vi "P2P_vst_ini.vi"(8 "error in (no error)":errorcluster, 11 "secnario config":T1={"devicess 2"=["IF_transiver_1", "IF_transiver_2"], "file paths"=[path "C:/Users/PXIe8108_Demo/Documents/CHAIM DATA/chaim/5785_sync_for_elbit/data/pdw_test_file.tdms", path "C:/Users/PXIe8108_Demo/Documents/CHAIM DATA/chaim/5785_sync_for_elbit/data/pdw_test_file.tdms", path "C:/Users/PXIe8108_Demo/Documents/CHAIM DATA/chaim/5785_sync_for_elbit/data/pdw_test_file.tdms", path "C:/Users/PXIe8108_Demo/Documents/CHAIM DATA/chaim/5785_sync_for_elbit/data/pdw_test_file.tdms"], "buffer size"=524288, "Fs  FPGA"=200000000.0, "SPC"=16.0, "center frequency (Hz) "=1000000000.0, "t clock ref"=[], "fpga rfe"=[], "tdms refs"=[], "niUsrpRio Session (out)"={"FPGA Interface"=refnum, "RIO Interface Number"=0, "Data Clock Rate"=0, "FPGA Data Clock Rate"=0, "Global Settings Register Bus"=refnum, "Radio 0 Settings Register Bus"=refnum, "Radio 1 Settings Register Bus"=refnum, "Radio Settings Bus Semaphore"=refnum, "DB Queues"=[], "Characterization Data Valid?"=FALSE, "EEPROM Header"={"Checksum"=0, "Product Code"=0, "Hardware Current Version"=0, "Hardware Oldest Compatible Version"=0, "EEPROM Map Current Version"=0, "EEPROM Map Oldest Compatible Version"=0, "User Password"="", "Pointer to Factory Header"=0, "Pointer to User Header"=0, "Recommended Interval"=0, "Number of Reserved Bytes"=9, "Number of Daughterboards"=0, "Daughterboard IDs"=[], "Daughterboard Serial Numbers"=[]}, "Device Data Header"={"Checksum"=0, "Number of Channels"=0, "Number of Gain Settings"=[], "Pointer to Characterization Data"=[], "Number of Reserved Bytes"=27, "Number of Frequencies"=[]}, "EEPROM Characterization Header"={"Checksum"=0, "Date"=timestamp(0 s since 1904-01-01), "Temperature"=0.0, "Misc. Info"="", "Pointer to Device Data Header"=0, "Number of Reserved Bytes"=28}, "Characterization Data"=[], "FPGA Current Version"=0, "FPGA Oldest Compatible Version"=0, "Fixed Logic Current Version"=0, "Fixed Logic Oldest Compatible Version"=0, "FPGA Radio Settings Bus Current Version"=0, "FPGA Radio Settings Bus Oldest Compatible Version"=0, "FPGA Board Config Current Version"=0, "FPGA Board Config Oldest Compatible Version"=0, "Daughterboard Clock Rate"=0, "daughterboard configuration session handles"=[]}, "RF gain "=10, "mode"=0, "vst_device"=[]} {"mode" scale=0.0..2.0; "RF gain" min=0 max=31 step=1; "niUsrpRio Session (out)"."Daughterboard Clock Rate" format="%#.3pHz"; "niUsrpRio Session (out)"."FPGA Data Clock Rate" format="%#.3pHz"; "niUsrpRio Session (out)"."Data Clock Rate" format="%#.3pHz"; "niUsrpRio Session (out)"."Characterization Data"."Frequencies [Hz]" format="%#_6p"; "niUsrpRio Session (out)"."EEPROM Characterization Header"."Pointer to Device Data Header" format="%x"; "niUsrpRio Session (out)"."EEPROM Characterization Header"."Checksum" format="%x"; "niUsrpRio Session (out)"."Device Data Header"."Pointer to Characterization Data" format="%x"; "niUsrpRio Session (out)"."Device Data Header"."Checksum" format="%x"; "niUsrpRio Session (out)"."EEPROM Header"."Pointer to User Header" format="%x"; "niUsrpRio Session (out)"."EEPROM Header"."Pointer to Factory Header" format="%x"; "niUsrpRio Session (out)"."EEPROM Header"."Product Code" format="%x"; "niUsrpRio Session (out)"."EEPROM Header"."Checksum" format="%x"; "center frequency (Hz)" format="%#.8p"; "buffer size" step=512}) -> (0 "error out":errorcluster, 3 "secnario config":T1={"devicess 2"=["IF_transiver_1", "IF_transiver_2"], "file paths"=[path "C:/Users/PXIe8108_Demo/Documents/CHAIM DATA/chaim/5785_sync_for_elbit/data/pdw_test_file.tdms", path "C:/Users/PXIe8108_Demo/Documents/CHAIM DATA/chaim/5785_sync_for_elbit/data/pdw_test_file.tdms", path "C:/Users/PXIe8108_Demo/Documents/CHAIM DATA/chaim/5785_sync_for_elbit/data/pdw_test_file.tdms", path "C:/Users/PXIe8108_Demo/Documents/CHAIM DATA/chaim/5785_sync_for_elbit/data/pdw_test_file.tdms"], "buffer size"=524288, "Fs  FPGA"=200000000.0, "SPC"=16.0, "center frequency (Hz) "=1000000000.0, "t clock ref"=[], "fpga rfe"=[], "tdms refs"=[], "niUsrpRio Session (out)"={"FPGA Interface"=refnum, "RIO Interface Number"=0, "Data Clock Rate"=0, "FPGA Data Clock Rate"=0, "Global Settings Register Bus"=refnum, "Radio 0 Settings Register Bus"=refnum, "Radio 1 Settings Register Bus"=refnum, "Radio Settings Bus Semaphore"=refnum, "DB Queues"=[], "Characterization Data Valid?"=FALSE, "EEPROM Header"={"Checksum"=0, "Product Code"=0, "Hardware Current Version"=0, "Hardware Oldest Compatible Version"=0, "EEPROM Map Current Version"=0, "EEPROM Map Oldest Compatible Version"=0, "User Password"="", "Pointer to Factory Header"=0, "Pointer to User Header"=0, "Recommended Interval"=0, "Number of Reserved Bytes"=9, "Number of Daughterboards"=0, "Daughterboard IDs"=[], "Daughterboard Serial Numbers"=[]}, "Device Data Header"={"Checksum"=0, "Number of Channels"=0, "Number of Gain Settings"=[], "Pointer to Characterization Data"=[], "Number of Reserved Bytes"=27, "Number of Frequencies"=[]}, "EEPROM Characterization Header"={"Checksum"=0, "Date"=timestamp(0 s since 1904-01-01), "Temperature"=0.0, "Misc. Info"="", "Pointer to Device Data Header"=0, "Number of Reserved Bytes"=28}, "Characterization Data"=[], "FPGA Current Version"=0, "FPGA Oldest Compatible Version"=0, "Fixed Logic Current Version"=0, "Fixed Logic Oldest Compatible Version"=0, "FPGA Radio Settings Bus Current Version"=0, "FPGA Radio Settings Bus Oldest Compatible Version"=0, "FPGA Board Config Current Version"=0, "FPGA Board Config Oldest Compatible Version"=0, "Daughterboard Clock Rate"=0, "daughterboard configuration session handles"=[]}, "RF gain "=10, "mode"=0, "vst_device"=[]} {"mode" scale=0.0..2.0; "RF gain" min=0 max=31 step=1; "niUsrpRio Session (out)"."Daughterboard Clock Rate" format="%#.3pHz"; "niUsrpRio Session (out)"."FPGA Data Clock Rate" format="%#.3pHz"; "niUsrpRio Session (out)"."Data Clock Rate" format="%#.3pHz"; "niUsrpRio Session (out)"."Characterization Data"."Frequencies [Hz]" format="%#_6p"; "niUsrpRio Session (out)"."EEPROM Characterization Header"."Pointer to Device Data Header" format="%x"; "niUsrpRio Session (out)"."EEPROM Characterization Header"."Checksum" format="%x"; "niUsrpRio Session (out)"."Device Data Header"."Pointer to Characterization Data" format="%x"; "niUsrpRio Session (out)"."Device Data Header"."Checksum" format="%x"; "niUsrpRio Session (out)"."EEPROM Header"."Pointer to User Header" format="%x"; "niUsrpRio Session (out)"."EEPROM Header"."Pointer to Factory Header" format="%x"; "niUsrpRio Session (out)"."EEPROM Header"."Product Code" format="%x"; "niUsrpRio Session (out)"."EEPROM Header"."Checksum" format="%x"; "center frequency (Hz)" format="%#.8p"; "buffer size" step=512})   [LabVIEW 2021]
uses:
  <vilib>/rvi/interface/nirviMethod/nirviMethod.xnode
  <vilib>/rvi/errors/niLvFpgaMergeErrorWithErrorCode.vi
  <vilib>/rvi/interface/nirviReadWriteControl/nirviReadWriteControl.xnode
  <vilib>/rvi/interface/nirviOpenFPGA/nirviOpenFPGA.xnode
  <instrlib>/niRFSG/niRFSG.llb/niRFSG Ref Clock Sources.ctl
  <instrlib>/niRFSG/niRFSG.llb/niRFSG Configure Start Trigger P2P Endpoint Fullness.vi
  <vilib>/FPGAPlugInAG/Dynamic/niLvFpga_StopFifo_Dynamic.vi
  <vilib>/FPGAPlugInAG/Dynamic/niLvFpga_ConfigureFifo_Dynamic.vi
  NiFpgaLv.dll
  <vilib>/Utility/error.llb/Error Cluster From Error Code.vi
  <vilib>/rvi/interface/Simulation/niFpgaSimulationCallBeginRW.vi
  <vilib>/rvi/errors/niLvFpgaAdjustHostInterfaceError.vi
  Users/PXIe8108_Demo/Documents/CHAIM DATA/chaim/5785_sync_for_elbit/tx_pulse/EMEA_ADG_EW_secnario_TX_PDW_to_pulses/FPGA Bitfiles/P2P_Pulse.lvbitx
  Users/PXIe8108_Demo/Documents/CHAIM DATA/chaim/5785_sync_for_elbit/tx_pulse/EMEA_ADG_EW_secnario_TX_PDW_to_pulses/fpga/5785_p2p_IQ_gen.vi
  <vilib>/FPGAPlugInAG/PXIe-5785 (KU060)/niLvFpga_Open_PXIe-5785 (KU060).vi
  <vilib>/rvi/interface/common/dynamic/niFpgaDynamicAddResources.vi
  <vilib>/userDefined/High Color/nirio_resource_hc.ctl
  secnario config.ctl
  Program Files/National Instruments/LabVIEW 2022/instr.lib/_niInstr/Register Bus/v0/Host/Private/Session Data.ctl
  Program Files/National Instruments/LabVIEW 2022/instr.lib/_niInstr/Register Bus/v0/Host/niInstr Register Bus v0 Host.lvlib
  Program Files/National Instruments/LabVIEW 2022/instr.lib/_niInstr/Register Bus/v0/Host/Public/Register Bus Session.ctl
  Program Files/National Instruments/LabVIEW 2022/instr.lib/niUsrpRio/Config/v1/Host/Public/EEPROM Header.ctl
  Program Files/National Instruments/LabVIEW 2022/instr.lib/niUsrpRio/Config/v1/Host/niUsrpRio Config v1 Host.lvlib
  Program Files/National Instruments/LabVIEW 2022/instr.lib/niUsrpRio/Config/v1/Host/Public/EEPROM Device Data Header.ctl
  Program Files/National Instruments/LabVIEW 2022/instr.lib/niUsrpRio/Config/v1/Host/Public/EEPROM Characterization Header.ctl
  Program Files/National Instruments/LabVIEW 2022/instr.lib/niUsrpRio/Config/v1/Host/Public/IQ Imbalance.ctl
  Program Files/National Instruments/LabVIEW 2022/instr.lib/niUsrpRio/Config/v1/Host/Public/Characterization Data.ctl
  Program Files/National Instruments/LabVIEW 2022/instr.lib/niUsrpRio/Config/v1/Host/Private/Antenna Configuration.ctl
  Program Files/National Instruments/LabVIEW 2022/instr.lib/niUsrpRio/Config/v1/Host/Private/ATR state data.ctl
  Program Files/National Instruments/LabVIEW 2022/instr.lib/niUsrpRio/Config/v1/Host/Private/CPLD Power Mode.ctl
  Program Files/National Instruments/LabVIEW 2022/instr.lib/niUsrpRio/Config/v1/Host/Private/Daughterboard Data.ctl
  Program Files/National Instruments/LabVIEW 2022/instr.lib/niUsrpRio/Config/v1/Host/Private/DB Queue Reference.ctl
  Program Files/National Instruments/LabVIEW 2022/instr.lib/niUsrpRio/Config/v1/Host/Public/niUsrpRio Session.ctl
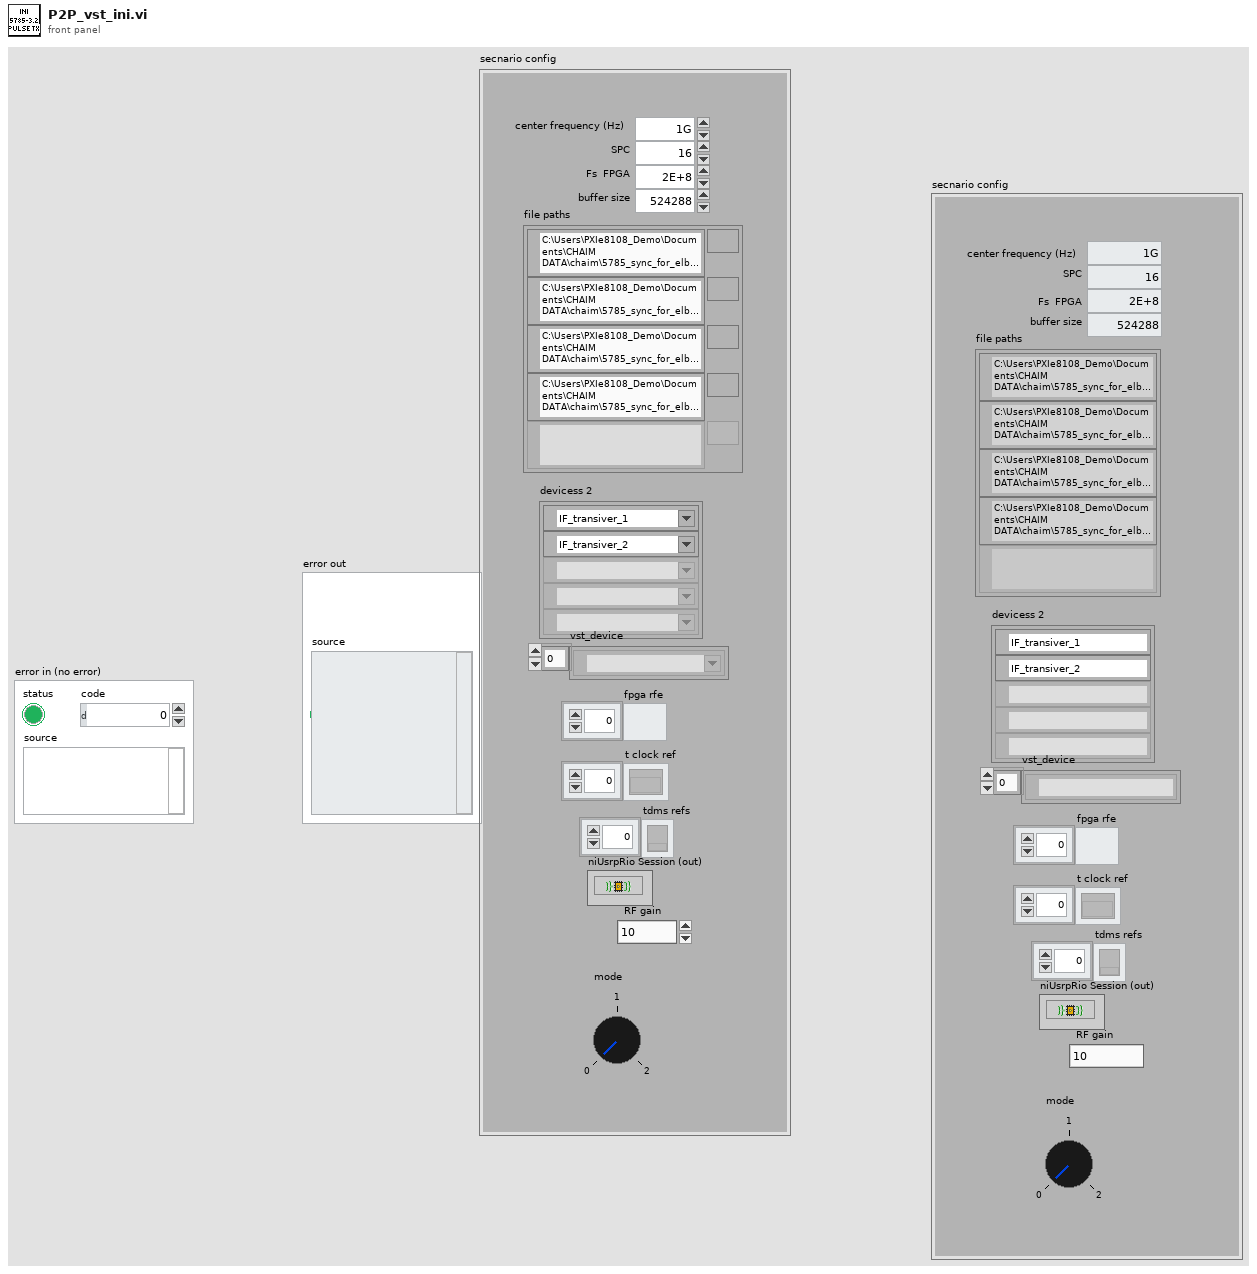
[diagram p1: front panel]
types:
  T1 = typedef "secnario config.ctl" = cluster{"devicess 2":T2[], "file paths":path[], "buffer size":u32, "Fs  FPGA":dbl, "SPC":dbl, "center frequency (Hz) ":dbl, "t clock ref":refnum<k20>[], "fpga rfe":refnum<k20>[], "tdms refs":refnum<k34>[], "niUsrpRio Session (out)":T3, "RF gain ":i32, "mode":u8, "vst_device":refnum<k15>[]}
  T2 = typedef "nirio_resource_hc.ctl" = tag
  T3 = typedef "niUsrpRio Config v1 Host.lvlib/niUsrpRio Session.ctl" = cluster{"FPGA Interface":refnum<k20>, "RIO Interface Number":u32, "Data Clock Rate":u32, "FPGA Data Clock Rate":u32, "Global Settings Register Bus":T4, "Radio 0 Settings Register Bus":T4, "Radio 1 Settings Register Bus":T4, "Radio Settings Bus Semaphore":T5, "DB Queues":T6[], "Characterization Data Valid?":bool, "EEPROM Header":T7, "Device Data Header":T8, "EEPROM Characterization Header":T9, "Characterization Data":T10[], "FPGA Current Version":u32, "FPGA Oldest Compatible Version":u32, "Fixed Logic Current Version":u32, "Fixed Logic Oldest Compatible Version":u32, "FPGA Radio Settings Bus Current Version":u32, "FPGA Radio Settings Bus Oldest Compatible Version":u32, "FPGA Board Config Current Version":u32, "FPGA Board Config Oldest Compatible Version":u32, "Daughterboard Clock Rate":u32, "daughterboard configuration session handles":u64[]}
  T4 = typedef "niInstr Register Bus v0 Host.lvlib/Register Bus Session.ctl" = refnum<queue>
  T5 = typedef "Semaphore RefNum" = refnum<k1>
  T6 = typedef "niUsrpRio Config v1 Host.lvlib/DB Queue Reference.ctl" = refnum<queue>
  T7 = typedef "niUsrpRio Config v1 Host.lvlib/EEPROM Header.ctl" = cluster{"Checksum":u32, "Product Code":u16, "Hardware Current Version":u16, "Hardware Oldest Compatible Version":u16, "EEPROM Map Current Version":u16, "EEPROM Map Oldest Compatible Version":u16, "User Password":string, "Pointer to Factory Header":u32, "Pointer to User Header":u32, "Recommended Interval":u16, "Number of Reserved Bytes":i32, "Number of Daughterboards":u8, "Daughterboard IDs":u16[], "Daughterboard Serial Numbers":string[]}
  T8 = typedef "niUsrpRio Config v1 Host.lvlib/EEPROM Device Data Header.ctl" = cluster{"Checksum":u32, "Number of Channels":u8, "Number of Gain Settings":u16[], "Pointer to Characterization Data":u32[], "Number of Reserved Bytes":i32, "Number of Frequencies":u16[]}
  T9 = typedef "niUsrpRio Config v1 Host.lvlib/EEPROM Characterization Header.ctl" = cluster{"Checksum":u32, "Date":timestamp, "Temperature":sgl, "Misc. Info":string, "Pointer to Device Data Header":u32, "Number of Reserved Bytes":i32}
  T10 = typedef "niUsrpRio Config v1 Host.lvlib/Characterization Data.ctl" = cluster{"Gains[dB]":dbl[], "Frequencies [Hz]":dbl[], "IQ Imbalance Table":T11[], "Measured Gains[dB]":dbl[][]}
  T11 = typedef "niUsrpRio Config v1 Host.lvlib/IQ Imbalance.ctl" = cluster{"Gain Imbalance [linear]":dbl, "Phase Imbalance [radians]":dbl, "Offset":cdb}
  T12 = typedef "niRFSG Ref Clock Sources.ctl" = string
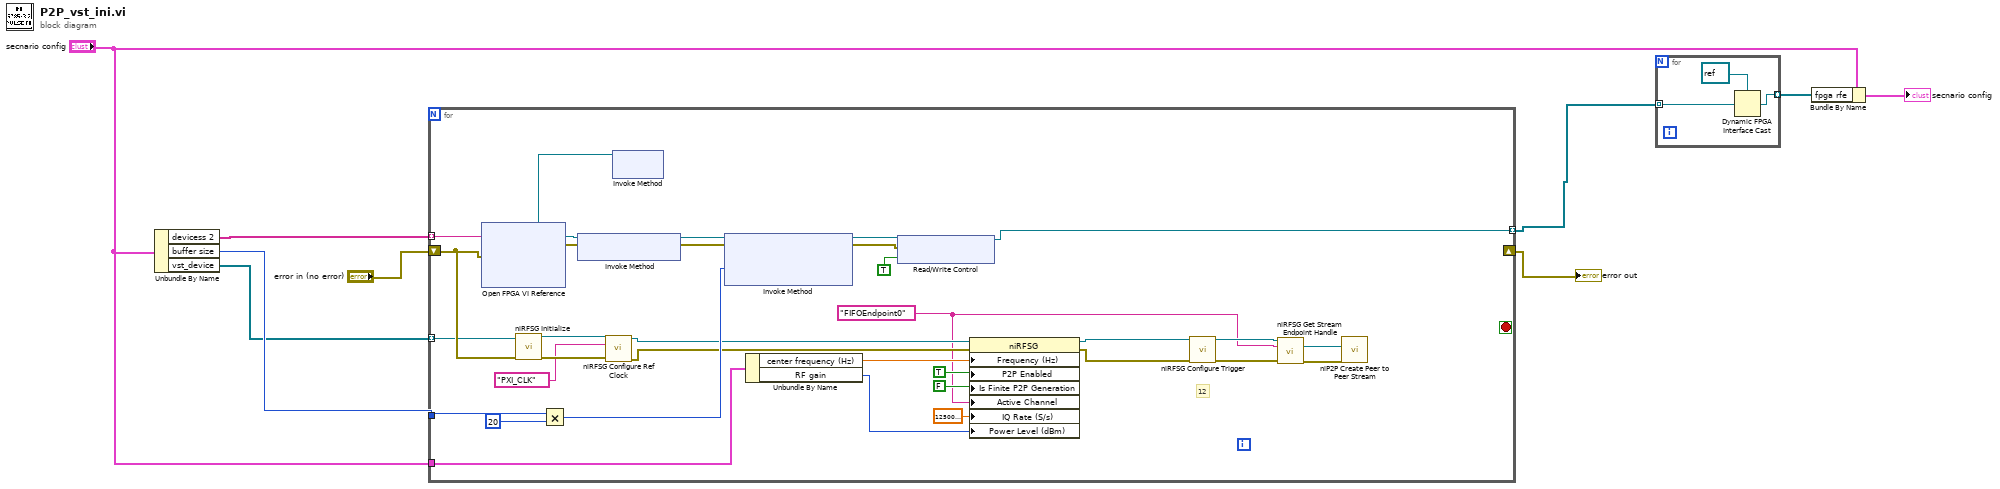
[diagram p0: block diagram]
diagram:
  n1 = Unbundle By Name("secnario config") -> ("devicess 2"=w7:T2[], "buffer size"=w6:u32, "vst_device"=w1:refnum<k15>[])
  n2 = for {
    tunnel: [w12] -> w5 mode=indexing
    shift-right: [_] -> w8
    shift-left: "error in (no error)" -> [w19]
    tunnel: w6 -> [w41]
    tunnel: w7 -> [w32] mode=indexing
    tunnel: "secnario config" -> [w26]
    tunnel: w1 -> [w10] mode=indexing
    stop <- _ stop-if-true
    w15 = "FIFOEndpoint0"
    # "12"
    n3 = xnode "Open FPGA VI Reference"("error in"=w19, "resource name"=w32) -> ("FPGA VI Reference Out"=w11:refnum<k20>, "error out"=w38:errorcluster)
    n4 = call <instrlib>:"niRFSG Initialize.vi"("resource name"=w10, "error in"=w19) -> ("instrument handle"=w31:refnum<k15>, "error out"=w30:errorcluster)  [unwired: 12 in]
    n5 = Multiply(x=w41, y=u32 20) -> (x*y=w40:u32)
    n6 = xnode "Invoke Method"("FPGA VI Reference In"=w11, "error in"=w38) -> ("FPGA VI Reference Out"=w36:refnum<k20>, "error out"=w37:errorcluster)
    n7 = call <instrlib>:"niRFSG Configure Ref Clock.vi"("instrument handle"=w31, "ref clock source"=T12 "PXI_CLK", "error in"=w30) -> ("instrument handle out"=w28:refnum<k15>, "error out"=w27:errorcluster)  [unwired: 11 in]
    n8 = xnode "Invoke Method"("FPGA VI Reference In"=w11) -> ()  [unwired: 1 in, 2 out]
    n9 = xnode "Invoke Method"("FPGA VI Reference In"=w36, "error in"=w37, "Requested Depth"=w40) -> ("FPGA VI Reference Out"=w34:refnum<k20>, "error out"=w33:errorcluster)  [unwired: 1 out]
    n10 = Unbundle By Name(w26) -> ("center frequency (Hz)"=w25:dbl, "RF gain"=w18:i32)
    n11 = xnode "Read/Write Control"("FPGA VI Reference In"=w34, "error in"=w33, "reset system clock"=TRUE) -> ("FPGA VI Reference Out"=w12:refnum<k20>)  [unwired: 1 out]
    n12 = property class="niRFSG"(reference=w28, error in=w27, "Frequency (Hz)"=w25, "P2P Enabled"=TRUE ("Peer-to-Peer:Enabled"), "Is Finite P2P Generation"=FALSE ("Peer-to-Peer:Is Finite Generation"), "Active Channel"=w15, "IQ Rate (S/s)"=1250000000.0 ("Arb:IQ Rate (S/s)"), "Power Level (dBm)"=w18) -> (reference out=w21:refnum<k15>, error out=w20:errorcluster)
    n13 = call-poly <instrlib>:"niRFSG Configure Trigger.vi"("instrument handle"=w21, "error in"=w20) -> ("instrument handle out"=w17:refnum<k15>, "error out"=w16:errorcluster)  [unwired: 12 in]
    n14 = call <instrlib>:"niRFSG Get Stream Endpoint Handle.vi"("instrument handle"=w17, "stream endpoint"=w15, "error in"=w16) -> ("reader handle"=w14:refnum<k20>, "error out"=w13:errorcluster)  [unwired: 10 in, 1 out]
    n15 = call <vilib>:"niP2P Create Peer to Peer Stream.vi"("reader"=w14, "error in (no error)"=w13) -> ()  [unwired: 12 in, 2 out]
  }
  "error out" <- w8
  n16 = for {
    tunnel: w5 -> [w43] mode=indexing
    tunnel: [w42] -> w4 mode=indexing
    n17 = Dynamic FPGA Interface Cast(Session In=refnum<k20> refnum ("fpga interface out"), Type=w43) -> (Session Out=w42:refnum<k20>)
  }
  n18 = Bundle By Name(cluster="secnario config", "fpga rfe"=w4) -> (→"secnario config":T1)
